vi "Drive Immediate.vi"(5 "Straight Setpoint":dbl, 7 "Description":string, 8 "Command Info In":T1, 9 "Deadband Value":dbl=0.01, 10 "Right Setpoint":dbl, 11 "Left Setpoint":dbl) -> (0 "Command Info Out":T1)   [LabVIEW 2015]
doc: "Often used for joystick control, this VI checks to see that the joystick axes are outside the deadband and updates the motors appropriately."
uses:
  <vilib>/Rock Robotics/WPI/Framework/Command Status Info.ctl
  <vilib>/Rock Robotics/WPI/Framework/Completion Status.ctl
  <vilib>/Rock Robotics/WPI/Framework/Completion Notifier.ctl
  Implementation/Drive Setpoints.ctl
  Implementation/Drive Operations.ctl
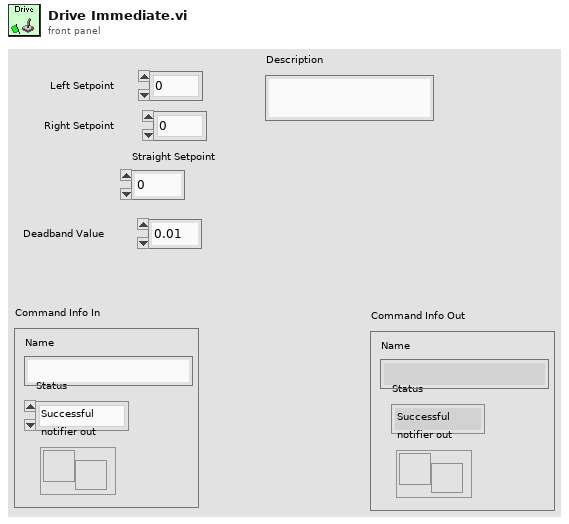
[diagram p1: front panel]
types:
  T1 = typedef "Command Status Info.ctl" = cluster{"Name":string, "Status":T2, "notifier out":T3}
  T2 = typedef "Completion Status.ctl" = enum16{"Successful", "Aborted", "Incomplete"}
  T3 = typedef "Completion Notifier.ctl" = refnum<notifier>
  T4 = typedef "Drive Setpoints.ctl" = cluster{"Operation":T5, "Left Setpoint":dbl, "Right Setpoint":dbl, "Duration":dbl, "Straight Setpoint":dbl}
  T5 = typedef "Drive Operations.ctl" = enum16{"Reserve", "Read Current", "Immediate", "Drive for Time", "Drive for Distance"}
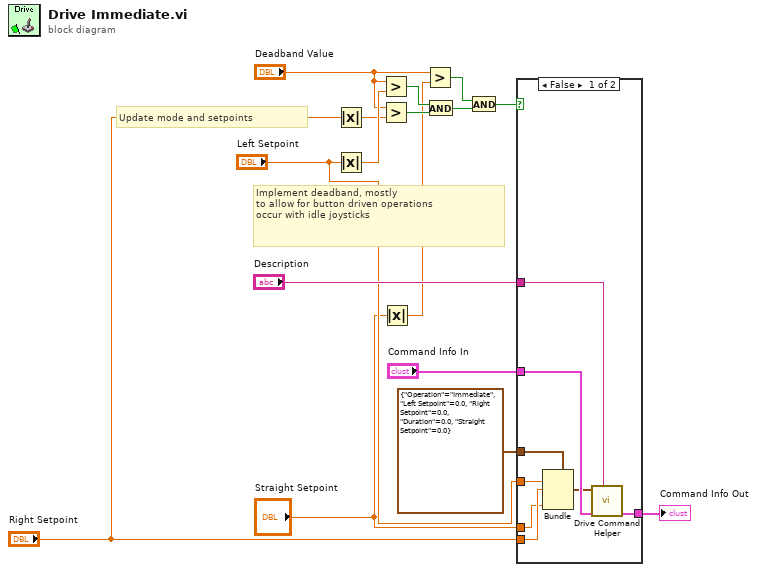
[diagram p0: block diagram]
diagram:
  # "Implement deadband, mostly\nto allow for button driven operations\noccur with idle joysticks"
  # "Update mode and setpoints"
  n1 = Absolute Value(x="Right Setpoint") -> (abs(x)=w8:dbl)
  n2 = Absolute Value(x="Left Setpoint") -> (abs(x)=w16:dbl)
  n3 = Greater?(x="Deadband Value", y=w16) -> (0:w10:bool)
  n4 = Greater?(x="Deadband Value", y=w8) -> (0:w6:bool)
  n5 = Absolute Value(x="Straight Setpoint") -> (abs(x)=w5:dbl)
  n6 = Greater?(x="Deadband Value", y=w5) -> (0:w1:bool)
  n7 = And(x=w10, y=w6) -> (x .and. y?=w9:bool)
  n8 = And(x=w1, y=w9) -> (x .and. y?=w2:bool)
  n9 = case shown="False" w2 {
    tunnel: "Left Setpoint" -> [w24 _]
    tunnel: T4 {"Operation"=enum."Immediate", "Left Setpoint"=0.0, "Right Setpoint"=0.0, "Duration"=0.0, "Straight Setpoint"=0.0} ("SubSystem Data") -> [w23 _]
    tunnel: [w22 w25] -> w15
    tunnel: "Command Info In" -> [w21 w25]
    tunnel: "Description" -> [w19 _]
    tunnel: "Right Setpoint" -> [w18 _]
    tunnel: "Straight Setpoint" -> [w17 _]
    frame False {
      n10 = Bundle(cluster=w23, "Left Setpoint"=w24, "Right Setpoint"=w18, "Straight Setpoint"=w17) -> (w20:T4)  [unwired: 2 in]
      n11 = call "Drive Command Helper.vi"("Description"=w19, "Command Info In"=w21, "SubSystem Data"=w20) -> ("Command Info Out"=w22:T1)  [unwired: 7 in, 1 out]
    }
    frame True {
    }
  }
  "Command Info Out" <- w15
